vi "MDOSave Configuration Settings to XML.vi"(8 "error in (no error)":errorcluster, 11 "User Configuration":T1 {"Hardware Configuration"."SyncMode" items=["INTERNAL"=0, "EXTERNAL_MASTER"=1, "DI_SYN1_RISE"=2, "DI_SYN1_FALL"=3, "DI_SYN2_RISE"=6, "DI_SYN2_FALL"=7]}) -> (0 "error out":errorcluster)   [LabVIEW 2012]
doc: "Saves the user-specified configuration data to an XML file. This is used to remember settings between executions."
uses:
  controls/MDOUser Specified Data.ctl
  controls/MDOHW Configuration.ctl
  controls/MDONew Data Behavior.ctl
  controls/Acquire_Type.ctl
  <vilib>/Utility/xml.llb/Write to XML File(string).vi
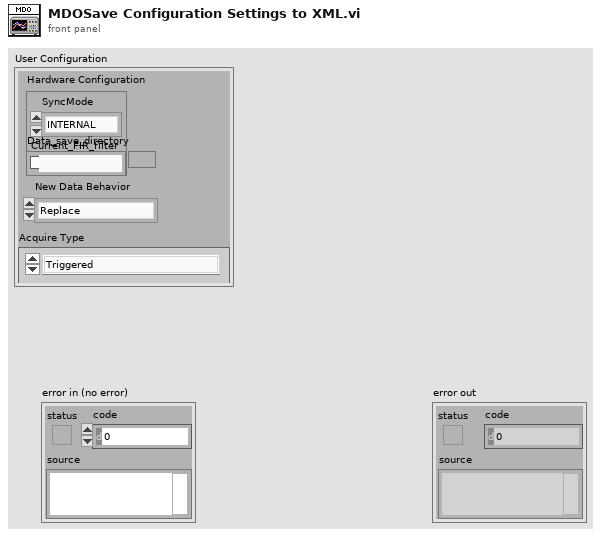
[diagram p1: front panel]
types:
  T1 = typedef "MDOUser Specified Data.ctl" = cluster{"Hardware Configuration":T2, "New Data Behavior":T3, "Acquire Type":T4, "Data_save_directory":path}
  T2 = typedef "MDOHW Configuration.ctl" = cluster{"SyncMode":u32, "Current_FIR_filter":bool}
  T3 = typedef "MDONew Data Behavior.ctl" = enum16{"Replace", "Overlay", "Append"}
  T4 = typedef "Acquire_Type.ctl" = enum16{"Triggered", "Continues"}
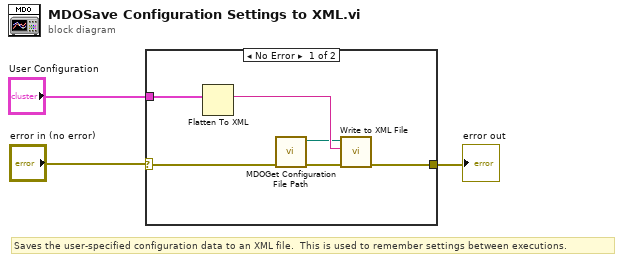
[diagram p0: block diagram]
diagram:
  # "Saves the user-specified configuration data to an XML file.  This is used to remember settings between executions."
  n1 = case shown="No Error" "error in (no error)" {
    selector: "error in (no error)" -> [w5 w10]
    tunnel: [w7 w10] -> w2
    tunnel: "User Configuration" -> [w9 _]
    frame No Error {
      n2 = Flatten To XML(anything=w9) -> (xml string=w8:string)
      n3 = call "MDOGet Configuration File Path.vi"("error in (no error)"=w5) -> ("error out"=w4:errorcluster, "XML File Path"=w6:path)  [unwired: 9 in]
      n4 = call-poly <vilib>:"Write to XML File.vi"("error in (no error)"=w4, "XML Input"=w8, "XML File Path"=w6) -> ("error out"=w7:errorcluster)  [unwired: 6 in, 2 out]
    }
    frame Error {
    }
  }
  "error out" <- w2
